vi "BuildTestFromProjectItem_Library_BuildsTestSuite.vi"() -> ()   [LabVIEW 2017, in "LVUnitTestBuilder.Tests.lvlib"]
uses:
  LVUnitTestBuilder.Tests.lvlib
  LVUnitTestBuilder/LVUnitTestBuilder.lvclass
  TestSuite/TestSuite.lvclass
  Assertion/Assertion.lvlib
panel:
  out "error out":errorcluster
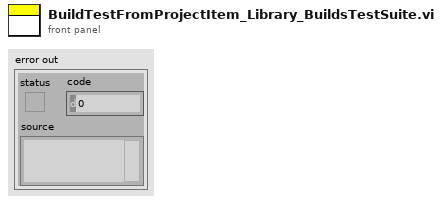
[diagram p1: front panel]
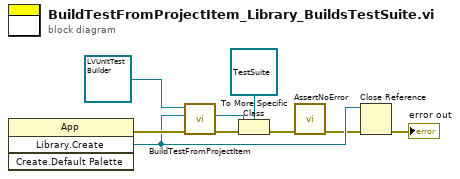
[diagram p0: block diagram]
diagram:
  n1 = invoke class="App" method="Library.Create"() -> (error out=w8:errorcluster, "Create Library"=w4:refnum<vi>)  [unwired: 4 in, 2 out]
  n2 = call-dynamic "BuildTestFromProjectItem.vi"("error in (no error)"=w8, "ProjectItem Refnum"=w4, "LVUnitTestBuilder in"=refnum<class "LVUnitTestBuilder.lvclass"> refnum ("LVUnitTestBuilder")) -> ("error out"=w3:errorcluster, "Test"=w7:refnum<class "Test.lvclass">)  [unwired: 6 in, 1 out]
  n3 = To More Specific Class(target class=refnum<class "TestSuite.lvclass"> refnum ("TestSuite.lvclass"), reference=w7, error in=w3) -> (error out=w2:errorcluster)  [unwired: 1 out]
  n4 = call "AssertNoError.vi"("error in (no error)"=w2) -> ("error out"=w1:errorcluster)  [unwired: 10 in]
  n5 = Close Reference(reference=w4, error in (no error)=w1) -> (error out=→"error out":errorcluster)
